vi "_iWorx - Spirometer.vi"() -> ()   [LabVIEW 2012]
uses:
  <vilib>/DAQmx/create/channels.llb/DAQmx Create Channel (AI-Voltage-Basic).vi
  <vilib>/DAQmx/read.llb/DAQmx Read (Analog 1D Wfm NChan 1Samp).vi
  <vilib>/DAQmx/configure/timing.llb/DAQmx Timing (Sample Clock).vi
  vi.lib/iWorx/iWorx Set Points.ctl
panel:
  in  "Reset Integral":bool=TRUE
  in  "Reset Scale":bool
  in  "Stop":bool
  in  "Log Info Button":bool
  in  "Set Up":bool
  in  "Channel":u16(ring) items=["Channel 1", "Channel 2"]
  in  "Pause Button":bool
  in  "Snapshot":bool
  out "Processed Signal":dbl(knob) caption="Pressue" scale=0.0..20.0
  out "Waveform Chart":waveform(dbl)[](graph)
  in  "Clear Chart":bool
  in  "Open Log":bool
  in  "Rescale Y":bool
  out "Raw Signal":dbl(knob) scale=-10.0..10.0
  # "iWorx - Spirometer - Data Logger"
  # "Sensor Input"
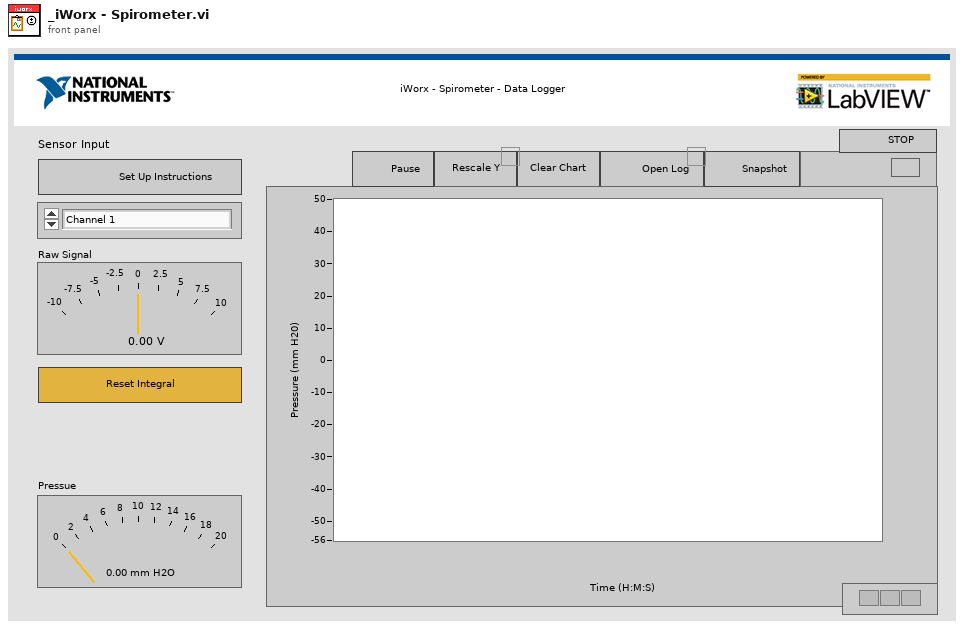
[diagram p1: front panel]
types:
  T1 = typedef "iWorx Set Points.ctl" = cluster{"SP1 Voltage":dbl, "SP1 Value":dbl, "SP2 Voltage":dbl, "SP2 Value":dbl}
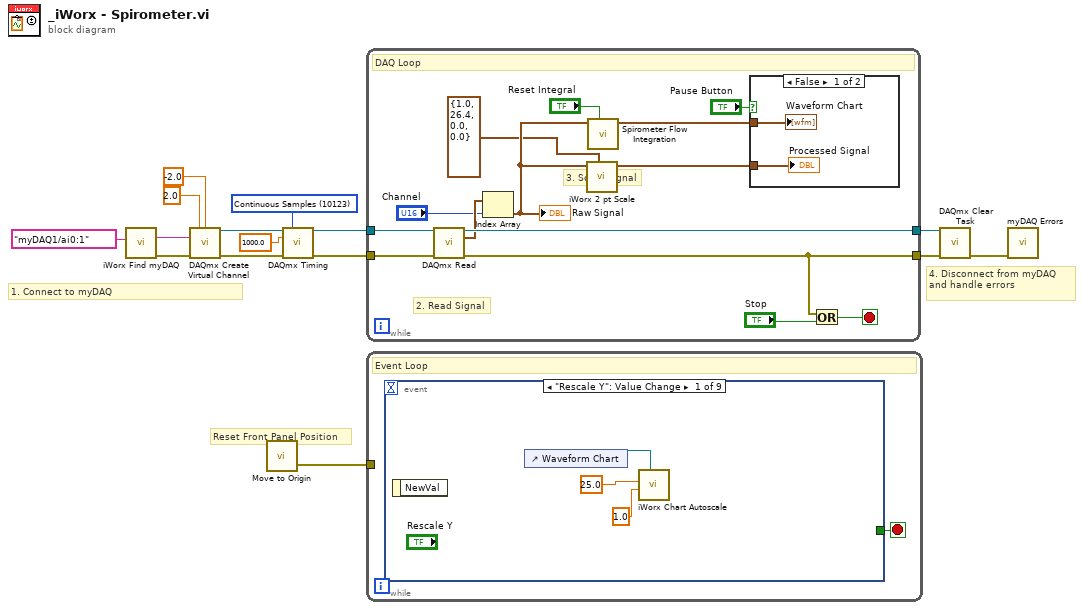
[diagram p0: block diagram]
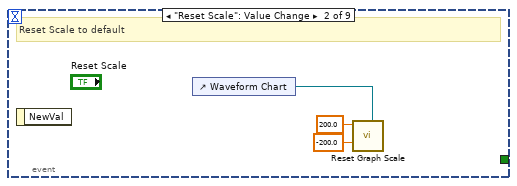
[diagram p2: hidden frame]
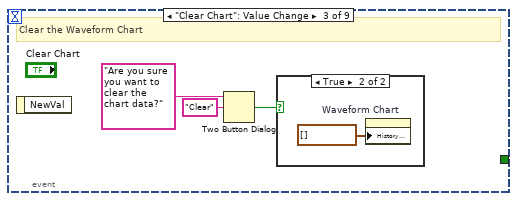
[diagram p3: hidden frame]
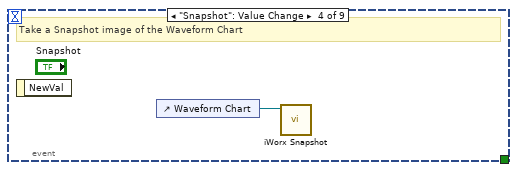
[diagram p5: hidden frame]
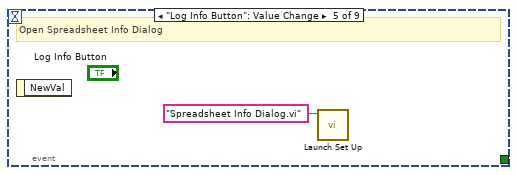
[diagram p6: hidden frame]
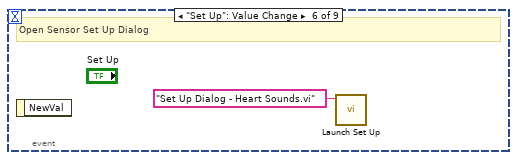
[diagram p7: hidden frame]
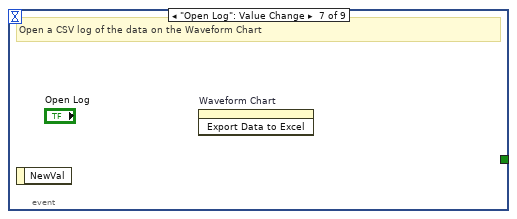
[diagram p8: hidden frame]
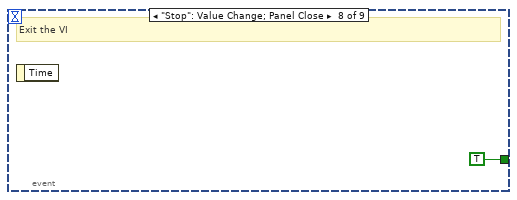
[diagram p9: hidden frame]
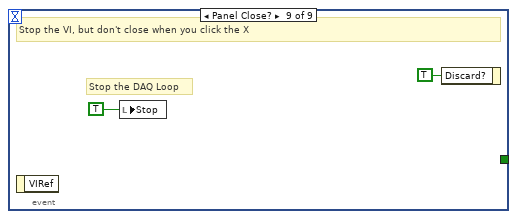
[diagram p10: hidden frame]
diagram:
  w6 = 10123 items=["Finite Samples"=10178, "Continuous Samples"=10123, "Hardware Timed Single Point"=12522] ("sample mode")
  # "Reset Front Panel Position"
  # "4. Disconnect from myDAQ and handle errors"
  # "1. Connect to myDAQ"
  n1 = call "iWorx Find myDAQ.vi"("Preferred myDAQ (myDAQ1)"=tag "myDAQ1/ai0:1") -> ("Error Out"=w11:errorcluster, "DAQmx Physical Channel"=w12:tag)  [unwired: 6 in, 3 out]
  n2 = call-poly <vilib>:"DAQmx Create Virtual Channel.vi"("maximum value"=2.0, "minimum value"=-2.0, "physical channels"=w12, "error in"=w11) -> ("task out"=w4:refnum<k21>, "error out"=w1:errorcluster)  [unwired: 10 in]
  n3 = call "Move to Origin.vi"() -> ("Error Out"=w9:errorcluster)  [unwired: 3 in]
  n4 = call-poly <vilib>:"DAQmx Timing.vi"("task/channels in"=w4, "sample mode"=w6, "rate"=1000.0, "error in"=w1) -> ("task out"=w3:refnum<k21>, "error out"=w2:errorcluster)  [unwired: 10 in]
  n5 = while {
    tunnel: w3 -> [w29]
    tunnel: [w28] -> w15
    tunnel: w2 -> [w27]
    tunnel: [w25] -> w14
    stop <- w26 stop-if-true
    # "3. Scale Signal"
    # "2. Read Signal"
    # "DAQ Loop"
    n6 = call-poly <vilib>:"DAQmx Read.vi"("task/channels in"=w29, "error in"=w27) -> ("task out"=w28:refnum<k21>, "data"=w23:waveform(dbl)[], "error out"=w25:errorcluster)  [unwired: 11 in]
    n7 = Index Array(array=w23, index="Channel") -> (element=w19:waveform(dbl))
    "Raw Signal" <- w19
    n8 = call "iWorx 2 pt Scale.vi"("Set Points"=T1 {"SP1 Voltage"=1.0, "SP1 Value"=26.4, "SP2 Voltage"=0.0, "SP2 Value"=0.0}, "Raw Waveform"=w19) -> ("Scaled Value"=w22:waveform(dbl))  [unwired: 7 in, 2 out]
    n9 = call "Spirometer Flow Integration.vi"("Reset Integral"="Reset Integral", "Waveform in"=w19) -> ("Waveform Array"=w18:waveform(dbl)[])  [unwired: 9 in]
    n10 = case shown="False" "Pause Button" {
      tunnel: w22 -> [w31 _]
      tunnel: w18 -> [w30 _]
      frame False {
        "Waveform Chart" <- w30
        "Processed Signal" <- w31
      }
      frame True {
        # "Do Not update controls"
      }
    }
    n11 = Or(x=w25, y="Stop") -> (x .or. y?=w26:bool)
  }
  n12 = while {
    tunnel: w9 -> [_]
    stop <- w32 stop-if-true
    # "Event Loop"
    n13 = event shown="[0] \"Rescale Y\": Value Change" {
      selector: _ -> [_ _ _ _ _ _ _ _ _]
      dyn-events: _ -> [_ _ _ _ _ _ _ _ _]
      timeout: _ -> [_ _ _ _ _ _ _ _ _]
      tunnel: [_ _ _ _ _ _ _ TRUE _] -> w32
      event "Rescale Y": Value Change {
        n14 = event-data() -> ()  [unwired: 1 in, 1 out]
        n15 = control-ref of="Waveform Chart"() -> (w33:refnum<vi>)
        n16 = call "iWorx Chart Autoscale.vi"("Selection Chart"=w33, "Rounding Multiple (10)"=1.0 ("Rounding Multiple (1)"), "Padding (10%)"=25.0 ("Rounding Multiple (1)")) -> ()  [unwired: 6 in, 3 out]
      }
      event "Reset Scale": Value Change {
        # "Reset Scale to default"
        n17 = event-data() -> ()  [unwired: 1 in, 1 out]
        n18 = control-ref of="Waveform Chart"() -> (w38:refnum<vi>)
        n19 = call "Reset Graph Scale.vi"("WaveformChart in"=w38, "Minimum (0)"=-200.0, "Maximum (100)"=200.0) -> ()  [unwired: 9 in]
      }
      event "Clear Chart": Value Change {
        # "Clear the Waveform Chart"
        n20 = event-data() -> ()  [unwired: 1 in, 1 out]
        n21 = Two Button Dialog(message="Are you sure you want to clear the chart data?", 2:"Clear" ("T button name (\"OK\")")) -> (T button?=w40:bool)  [unwired: 1 in]
        n22 = case shown="True" w40 {
          frame False {
          }
          frame True {
            n23 = property on="Waveform Chart" class="WFChart (strict)"("History Data"=waveform(dbl)[] []) -> ()  [unwired: 2 in, 2 out]
          }
        }
      }
      event "Snapshot": Value Change {
        # "Take a Snapshot image of the Waveform Chart"
        n24 = event-data() -> ()  [unwired: 1 in, 1 out]
        n25 = control-ref of="Waveform Chart"() -> (w43:refnum<vi>)
        n26 = call "iWorx Snapshot.vi"("WaveformChart in"=w43) -> ()  [unwired: 10 in, 1 out]
      }
      event "Log Info Button": Value Change {
        # "Open Spreadsheet Info Dialog"
        n27 = event-data() -> ()  [unwired: 1 in, 1 out]
        n28 = call "Launch Set Up.vi"("name or relative path"="Spreadsheet Info Dialog.vi") -> ()  [unwired: 9 in, 2 out]
      }
      event "Set Up": Value Change {
        # "Open Sensor Set Up Dialog"
        n29 = event-data() -> ()  [unwired: 1 in, 1 out]
        n30 = call "Launch Set Up.vi"("name or relative path"="Set Up Dialog - Heart Sounds.vi") -> ()  [unwired: 9 in, 2 out]
      }
      event "Open Log": Value Change {
        # "Open a CSV log of the data on the Waveform Chart"
        n31 = event-data() -> ()  [unwired: 1 in, 1 out]
        n32 = invoke on="Waveform Chart" class="WFChart (strict)" method="Export Data to Excel"() -> ()  [unwired: 3 in, 3 out]
      }
      event "Stop": Value Change; Panel Close {
        # "Exit the VI"
        n33 = event-data() -> ()  [unwired: 1 in, 1 out]
      }
      event Panel Close? {
        # "Stop the DAQ Loop"
        # "Stop the VI, but don't close when you click the X"
        n34 = event-data() -> ()  [unwired: 1 in, 1 out]
        n35 = local write "Stop"(TRUE ("stop")) -> ()
        n36 = event-data("Discard?"=TRUE) -> ()  [unwired: 1 in, 1 out]
      }
    }
  }
  n37 = call <vilib>:"DAQmx Clear Task.vi"("task in"=w15, "error in"=w14) -> ("error out"=w13:errorcluster)  [unwired: 13 in]
  n38 = call "myDAQ Errors.vi"("error in (no error)"=w13) -> ()  [unwired: 10 in, 1 out]
